vi "Radians to Degrees.vi"   [LabVIEW 2017, in "NI_AngleManipulation.lvlib"]
doc: "Converts an angle from radians to degrees."
uses:
  <vilib>/Utility/AngleManip/NI_AngleManipulation.lvlib
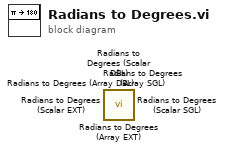
[diagram p0: block diagram]
diagram:
  n1 = call <vilib>:"Radians to Degrees (Array EXT).vi"() -> ()  [unwired: 3 in, 1 out]
  n2 = call <vilib>:"Radians to Degrees (Array SGL).vi"() -> ()  [unwired: 3 in, 1 out]
  n3 = call <vilib>:"Radians to Degrees (Scalar EXT).vi"() -> ()  [unwired: 3 in, 1 out]
  n4 = call <vilib>:"Radians to Degrees (Scalar SGL).vi"() -> ()  [unwired: 3 in, 1 out]
  n5 = call <vilib>:"Radians to Degrees (Array DBL).vi"() -> ()  [unwired: 3 in, 1 out]
  n6 = call <vilib>:"Radians to Degrees (Scalar DBL).vi"() -> ()  [unwired: 3 in, 1 out]
